vi "ALR init enums.vi"(7 "KFM_fcode_full":string[](array[string]), 8 "error in (no error)":errorcluster, 9 "DI_fcode_full":string[](array[string]), 10 "AI_fcode_full":string[](array[string]), 11 "Alarms in":T1) -> (0 "error":errorcluster, 3 "Alarms out":T1)   [LabVIEW 2019, in "Alarms.lvlib"]
uses:
  Alarms.lvlib
  Ctl/Alarms.ctl
  Ctl/ALR_defs.ctl
  Ctl/ALRs_State.ctl
  Ctl/ALR_ON_OFF.ctl
  Ctl/ALR_Parameters.ctl
  Ctl/ALR code.ctl
  Ctl/ALR type.ctl
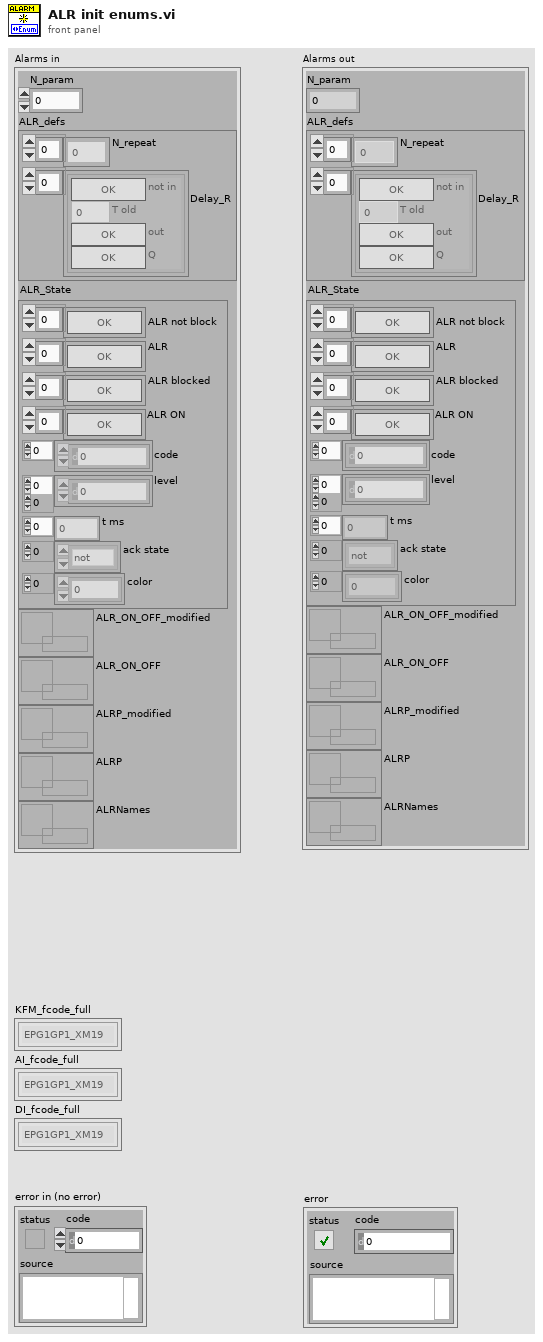
[diagram p1: front panel]
types:
  T1 = typedef "Alarms.lvlib/Alarms.ctl" = cluster{"N_param":i32, "ALR_defs":T2, "ALR_State":T3, "ALR_ON_OFF_modified":refnum<data-value>, "ALR_ON_OFF":refnum<data-value>, "ALRP_modified":refnum<data-value>, "ALRP":refnum<data-value>, "ALRNames":refnum<data-value>}
  T2 = typedef "Alarms.lvlib/ALR_defs.ctl" = cluster{"N_repeat":u32[], "Delay_R":cluster{"not in":bool, "T old":u32, "out":bool, "Q":bool}[]}
  T3 = typedef "Alarms.lvlib/ALRs_State.ctl" = cluster{"ALR not block":bool[], "ALR":bool[], "ALR blocked":bool[], "ALR ON":bool[], "code":i32[], "level":i32[][], "t ms":u32[], "ack state":enum32{"not", "tripped", "reset", "ack"}[], "color":u32[]}
  T4 = typedef "Alarms.lvlib/ALR_Parameters.ctl" = cluster{"ALR code":T5[], "ALR type":T6[], "ALRParam":u32[][]}
  T5 = typedef "Alarms.lvlib/ALR code.ctl" = enum16{"CONN", "H", "HH", "L", "LL", "SERR", "ON", "OFF", "XM19", "XM24", "XM47", "XM51", "XM52", "XM53", "XM54", "XM55", "XM56", "XM61", "XM62", "XM63", "XM64", "XM65", "XM66"}
  T6 = typedef "Alarms.lvlib/ALR type.ctl" = enum16{"ACD", "ACDR", "ALRN", "ALR"}
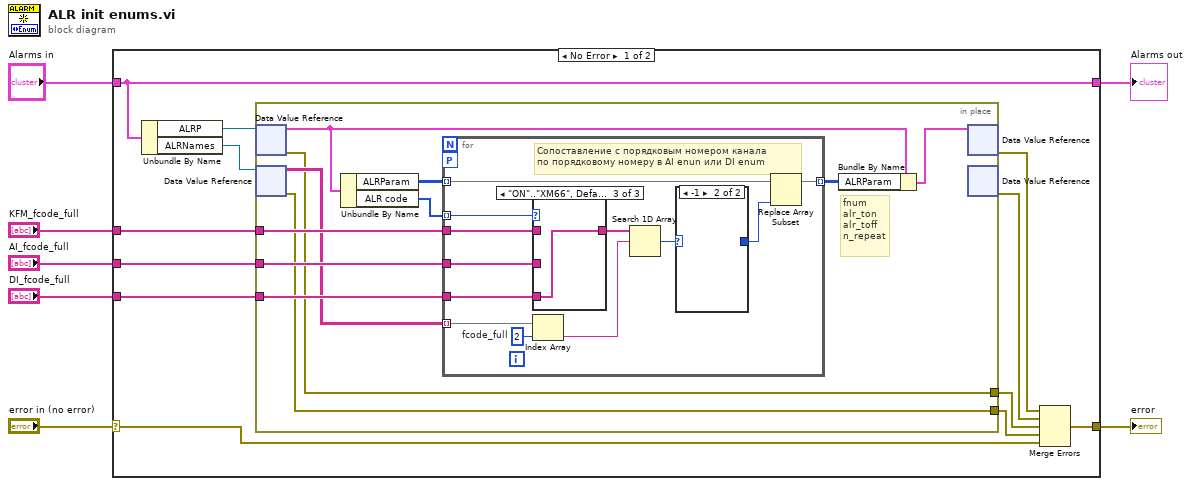
[diagram p0: block diagram]
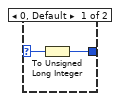
[diagram p2: hidden frame]
diagram:
  n1 = case shown="No Error" "error in (no error)" {
    selector: "error in (no error)" -> [w10 w49]
    tunnel: [w8 w49] -> w7
    tunnel: "Alarms in" -> [w9 w48]
    tunnel: "DI_fcode_full" -> [w19 _]
    tunnel: "AI_fcode_full" -> [w18 _]
    tunnel: [w9 w48] -> w2
    tunnel: "KFM_fcode_full" -> [w17 _]
    frame No Error {
      n2 = Unbundle By Name(w9) -> ("ALRP"=w15:refnum<data-value>, "ALRNames"=w16:refnum<data-value>)
      n3 = in-place {
        in-place-border: w19 -> [w30]
        in-place-border: w18 -> [w29]
        in-place-border: w17 -> [w28]
        in-place-border: [w21] -> w12
        in-place-border: [w20] -> w11
        # "fnum\nalr_ton\nalr_toff\nn_repeat"
        n4 = in-place-dvr #1(w15) -> (w23:T4, w21:errorcluster)
        n5 = in-place-dvr #2(w16) -> (w27:string[][], w20:errorcluster)
        n6 = Unbundle By Name(w23) -> ("ALRParam"=w25:u32[][], "ALR code"=w26:T5[])
        n7 = for {
          tunnel: w26 -> [w40] mode=indexing
          tunnel: w30 -> [w42]
          tunnel: w29 -> [w41]
          tunnel: w27 -> [w37] mode=indexing
          workers-P: _ -> [_]
          tunnel: w25 -> [w39] mode=indexing
          tunnel: [w38] -> w24 mode=indexing
          tunnel: w28 -> [w34]
          w36 = 2  # fcode_full
          # "Сопоставление с порядковым номером канала\nпо порядковому номеру в AI enun или DI enum"
          n8 = case shown="\"ON\"..\"XM66\", Default" w40 {
            tunnel: w42 -> [_ _ w47]
            tunnel: w41 -> [_ w46 _]
            tunnel: w34 -> [w45 _ _]
            tunnel: [w45 w46 w47] -> w32
            frame "CONN" {
            }
            frame "H".."SERR" {
            }
            frame "ON".."XM66", Default {
            }
          }
          n9 = Index Array(array=w37, index=w36) -> (element=w31:string)
          n10 = Search 1D Array(1D array=w32, element=w31) -> (index of element=w33:i32)  [unwired: 1 in]
          n11 = case shown="-1" w33 {
            selector: w33 -> [w43 _]
            tunnel: [w44 _] -> w35
            frame 0, Default {
              n12 = To Unsigned Long Integer(number=w43) -> (unsigned 32bit integer=w44:u32)
            }
            frame -1 {
            }
          }
          n13 = Replace Array Subset(array=w39, new element=w35) -> (w38:u32[])  [unwired: 1 in]
        }
        n14 = Bundle By Name(cluster=w23, "ALRParam"=w24) -> (w22:T4)
        n15 = in-place-dvr #1(w22) -> (w14:errorcluster)  [unwired: 1 out]
        n16 = in-place-dvr #2() -> (w13:errorcluster)  [unwired: 1 in, 1 out]
      }
      n17 = Merge Errors(w14, w13, w12, w11, w10) -> (w8:errorcluster)
    }
    frame Error {
    }
  }
  "error" <- w7
  "Alarms out" <- w2
